vi "Create Cluster Of Simple Arithmetic Class Instance.vi"() -> (3 "Cluster With Class":T1)   [LabVIEW 2012]
uses:
  ClassDefinitions/SimpleClassWithMethods/SimpleArithmetic.lvclass
panel:
  in  "Numeric":dbl
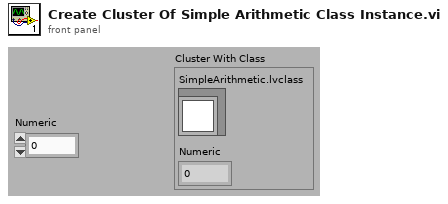
[diagram p1: front panel]
types:
  T1 = cluster{"SimpleArithmetic.lvclass":refnum<class "SimpleArithmetic.lvclass">, "Numeric":dbl}
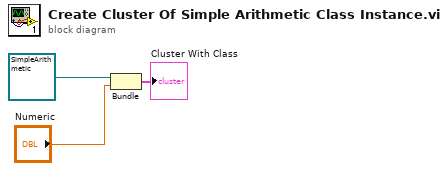
[diagram p0: block diagram]
diagram:
  n1 = Bundle("SimpleArithmetic.lvclass"=refnum<class "SimpleArithmetic.lvclass"> refnum, "Numeric"="Numeric") -> (→"Cluster With Class":T1)  [unwired: 1 in]
